vi "מסך ייצור 2 8.11.vi"(1 "Order":string[](array[string])) -> ()   [LabVIEW 2013]
uses:
  <vilib>/Utility/file.llb/Read From Spreadsheet File (string).vi
  Global 3.vi
  <vilib>/Utility/file.llb/Write To Spreadsheet File (string).vi
panel:
  out "element 2":string
  out "element":string
  out "row":i32
  out "output string":string
  out "decimal integer string":string[](array[string])
  out "size(s)":i32[](array[numeric])
  in  "v ok":bool
  out "Boolean 7":bool
  out "Boolean 6":bool
  out "Boolean 8":bool
  out "orders":string[][](array[string])
  out "int 9":dbl
  out "N itertion 9":dbl
  out "x/y 9":dbl
  out "int 8":dbl
  out "N itertion 8":dbl
  out "x/y 8":dbl
  out "x/y 7":dbl
  out "N itertion 7":dbl
  out "int 7":dbl
  out "int 6":dbl
  out "N itertion 6":dbl
  out "x/y 6":dbl
  out "int 5":dbl
  out "N itertion 5":dbl
  out "x/y 5":dbl
  out "x/y 4":dbl
  out "N itertion 4":dbl
  out "int 4":dbl
  out "Boolean 5":bool
  out "Boolean 4":bool
  out "Boolean 3":bool
  out "Boolean 2":bool
  out "Boolean":bool
  out "ML INT":dbl
  out "x/y 3":dbl
  out "N itertion 3":dbl
  out "int 3":dbl
  out "x/y 2":dbl
  out "N itertion 2":dbl
  out "int 2":dbl
  out "int":dbl
  out "N itertion":dbl
  out "x/y":dbl
  out "camot":dbl
  out "CAMOT":string
  out "ML":string
  out "Virus C":dbl(slide) scale=0.0..80.0
  out "Virus B":dbl(slide) scale=0.0..80.0
  out "Virus A":dbl(slide) scale=0.0..80.0
  out "HISON":string
  in  "EXIT":bool
  out "bottels ready":dbl(slide)
  out "Production Tank":dbl(slide) scale=0.0..100.0
  in  "start":bool
  out "Water":dbl(slide) scale=0.0..50.0
  out "Classifier material":dbl(slide) scale=0.0..25.0
  out "status":string
  # "Fider"
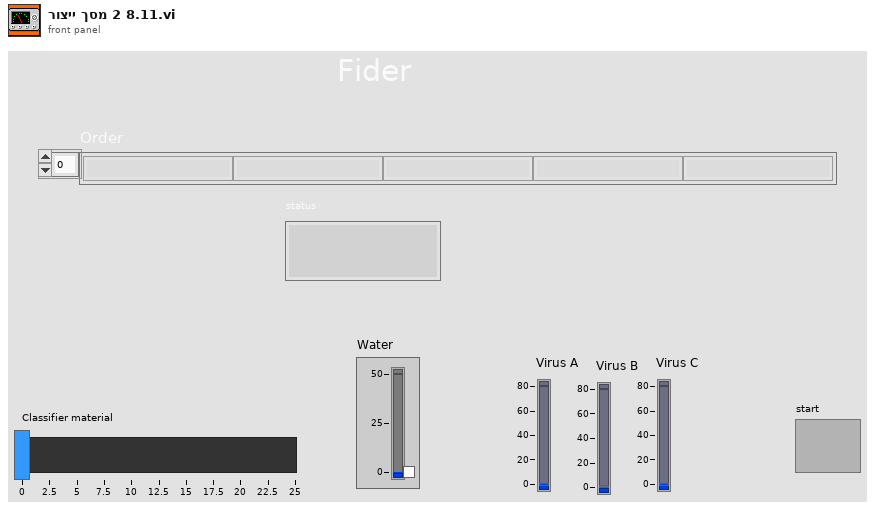
[diagram p1: front panel]
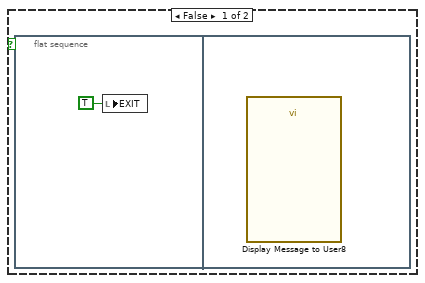
[diagram p3: hidden frame]
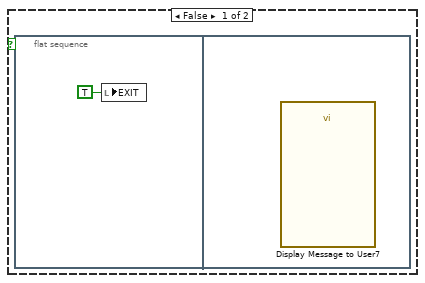
[diagram p5: hidden frame]
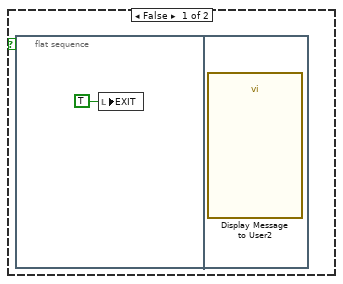
[diagram p7: hidden frame]
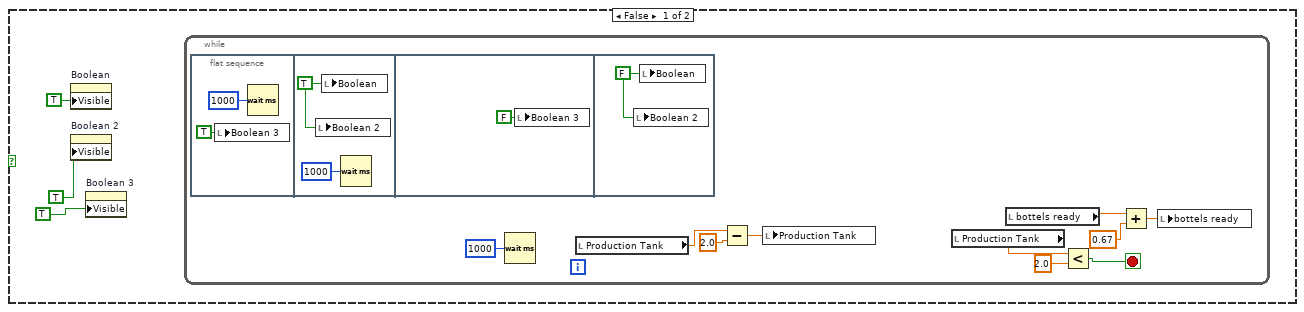
[diagram p10: hidden frame]
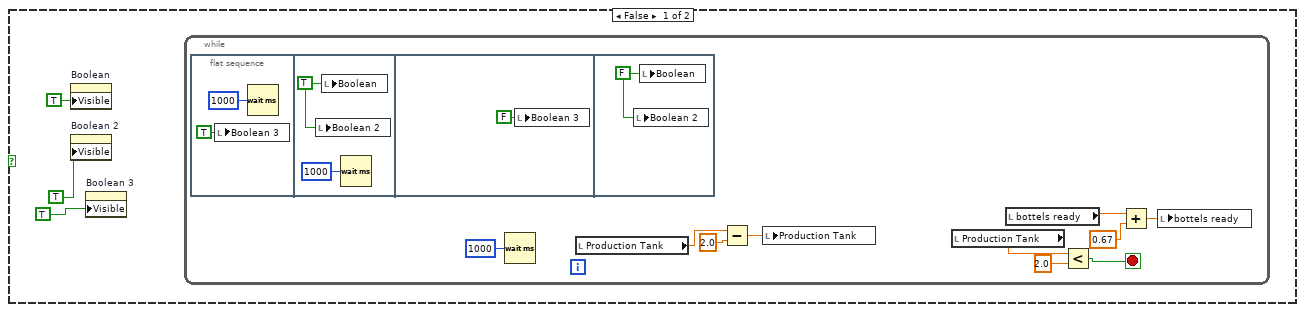
[diagram p12: hidden frame]
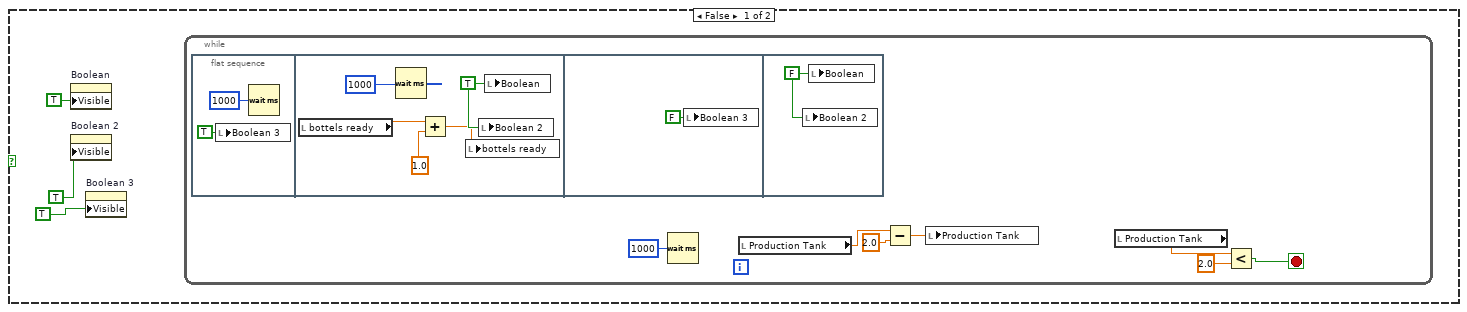
[diagram p14: hidden frame]
diagram:
  n1 = flat-sequence {
    frame #0 {
      n2 = local write "v ok"(FALSE ("v ok")) -> ()
      n3 = local write "EXIT"(FALSE ("EXIT")) -> ()
      n4 = local write "start"(FALSE ("start")) -> ()
    }
    frame #1 {
      n5 = while {
        stop <- "EXIT" stop-if-true
        n6 = local read "Order"() -> (w42:string[])
        n7 = property on="Classifier material" class="Slide (strict)"("Visible"=TRUE) -> ()  [unwired: 2 in, 2 out]
        n8 = global read "Global 3.vi" "Virus C"() -> (→"Virus C":dbl)
        n9 = property on="Boolean 4" class="Bool (strict)"("Visible"=FALSE) -> ()  [unwired: 2 in, 2 out]
        n10 = property on="Boolean" class="Bool (strict)"("Visible"=FALSE) -> ()  [unwired: 2 in, 2 out]
        n11 = property on="Boolean 2" class="Bool (strict)"("Visible"=FALSE) -> ()  [unwired: 2 in, 2 out]
        n12 = property on="Boolean 5" class="Bool (strict)"("Visible"=FALSE) -> ()  [unwired: 2 in, 2 out]
        n13 = property on="Boolean 3" class="Bool (strict)"("Visible"=FALSE) -> ()  [unwired: 2 in, 2 out]
        n14 = local read "Order"() -> (w41:string[])
        n15 = property on="Production Tank" class="Slide (strict)"("Blinking"=FALSE) -> ()  [unwired: 2 in, 2 out]
        n16 = property on="Production Tank" class="Slide (strict)"("Visible"=FALSE) -> ()  [unwired: 2 in, 2 out]
        n17 = Index Array(array=w42, index=2) -> (element=→"HISON":string)
        n18 = property on="bottels ready" class="Slide (strict)"("Visible"=FALSE) -> ()  [unwired: 2 in, 2 out]
        n19 = property on="Water" class="Slide (strict)"("Visible"=TRUE) -> ()  [unwired: 2 in, 2 out]
        n20 = global read "Global 3.vi" "Virus B"() -> (→"Virus B":dbl)
        n21 = local read "decimal integer string"() -> (w7:string[])
        n22 = Index Array(array=w41, index=4) -> (element=→"CAMOT":string)
        n23 = property on="Virus A" class="Slide (strict)"("Visible"=TRUE) -> ()  [unwired: 2 in, 2 out]
        n24 = property on="Virus B" class="Slide (strict)"("Visible"=TRUE) -> ()  [unwired: 2 in, 2 out]
        n25 = local read "Order"() -> (w40:string[])
        n26 = Current VI's Path() -> (path=w18:path)
        n27 = local read "orders"() -> (w10:string[][])
        n28 = property on="Virus C" class="Slide (strict)"("Visible"=TRUE) -> ()  [unwired: 2 in, 2 out]
        n29 = Strip Path(path=w18) -> (stripped path=w17:path)  [unwired: 1 out]
        n30 = local read "CAMOT"() -> (w22:string)
        n31 = global read "Global 3.vi" "Virus A"() -> (→"Virus A":dbl)
        n32 = global read "Global 3.vi" "Classifier material"() -> (→"Classifier material":dbl)
        n33 = Index String Array(1:0 ("index"), 2:w7) -> (0:w5:string)  [unwired: 1 in]
        "output string" <- w5
        n34 = local read "camot"() -> (w21:dbl)
        n35 = Index Array(array=w40, index=3) -> (element=→"ML":string)
        n36 = Build Path(base path=w17, name or relative path="order list.xls") -> (appended path=w16:path)
        n37 = Array Size(array=w10) -> (size(s)=w9:i32[])
        "size(s)" <- w9
        n38 = Fract/Exp String To Number(string=w22) -> (number=→"camot":dbl)  [unwired: 3 in, 1 out]
        n39 = global read "Global 3.vi" "Water"() -> (→"Water":dbl)
        n40 = Decimal String To Number(string=w5) -> (number=→"row":i32)  [unwired: 2 in, 1 out]
        n41 = property on="bottels ready" class="Slide (strict)"("Scale.Maximum"=w21) -> ()  [unwired: 2 in, 2 out]
        n42 = call-poly <vilib>:"Read From Spreadsheet File.vi"("file path (dialog if empty)"=w16) -> ("all rows"=→"orders":string[][])  [unwired: 6 in, 4 out]
        n43 = local read "ML"() -> (w39:string)
        n44 = Number To Decimal String(number=w9) -> (decimal integer string=→"decimal integer string":string[])  [unwired: 1 in]
        n45 = Fract/Exp String To Number(string=w39) -> (number=→"ML INT":dbl)  [unwired: 3 in, 1 out]
        n46 = flat-sequence {
          frame #0 {
            n47 = local read "HISON"() -> (w59:string)
            n48 = local read "HISON"() -> (w57:string)
            n49 = Equal?(x=w59, y="Jaundice") -> (x = y?=w60:bool)
            n50 = local read "HISON"() -> (w54:string)
            n51 = case shown="True" w60 {
              frame False {
              }
              frame True {
                n52 = local read "ML INT"() -> (w76:dbl)
                n53 = local read "ML INT"() -> (w71:dbl)
                n54 = local read "ML INT"() -> (w68:dbl)
                n55 = local read "Classifier material"() -> (w81:dbl)
                n56 = local read "Virus C"() -> (w83:dbl)
                n57 = local read "Water"() -> (w82:dbl)
                n58 = Multiply(x=w76, y=0.08) -> (x*y=w77:dbl)
                n59 = Multiply(x=w71, y=0.9) -> (x*y=w70:dbl)
                n60 = Multiply(x=w68, y=0.02) -> (x*y=w69:dbl)
                n61 = local read "camot"() -> (w74:dbl)
                n62 = local read "camot"() -> (w73:dbl)
                n63 = local read "camot"() -> (w66:dbl)
                n64 = Multiply(x=w74, y=w77) -> (x*y=w78:dbl)
                n65 = Greater Or Equal?(x=w81, y=w78) -> (x >= y?=w62:bool)
                n66 = Multiply(x=w73, y=w70) -> (x*y=w79:dbl)
                n67 = Greater Or Equal?(x=w82, y=w79) -> (x >= y?=w63:bool)
                n68 = Multiply(x=w66, y=w69) -> (x*y=w80:dbl)
                n69 = And(x=w62, y=w63) -> (x .and. y?=w64:bool)
                n70 = Greater Or Equal?(x=w83, y=w80) -> (x >= y?=w65:bool)
                n71 = And(x=w64, y=w65) -> (x .and. y?=w61:bool)
                n72 = case shown="True" w61 {
                  frame False {
                    n73 = flat-sequence {
                      frame #0 {
                        n74 = local write "EXIT"(TRUE ("EXIT")) -> ()
                      }
                      frame #1 {
                        n75 = call "Display Message to User8"() -> ()  [unwired: 10 in, 2 out]
                      }
                    }
                  }
                  frame True {
                    n76 = property on="start" class="Bool (strict)"("Visible"=TRUE) -> ()  [unwired: 2 in, 2 out]
                    "Boolean 8" <- TRUE ("Boolean 6")
                  }
                }
              }
            }
            n77 = Equal?(x=w57, y="Influenza") -> (x = y?=w58:bool)
            n78 = case shown="True" w58 {
              frame False {
              }
              frame True {
                n79 = local read "ML INT"() -> (w104:dbl)
                n80 = local read "ML INT"() -> (w99:dbl)
                n81 = local read "Classifier material"() -> (w107:dbl)
                n82 = local read "ML INT"() -> (w93:dbl)
                n83 = Multiply(x=w104, y=0.81) -> (x*y=w105:dbl)
                n84 = Multiply(x=w99, y=0.15) -> (x*y=w100:dbl)
                n85 = local read "camot"() -> (w102:dbl)
                n86 = local read "camot"() -> (w97:dbl)
                n87 = local read "Virus B"() -> (w109:dbl)
                n88 = local read "camot"() -> (w95:dbl)
                n89 = Multiply(x=w102, y=w105) -> (x*y=w106:dbl)
                n90 = Multiply(x=w97, y=w100) -> (x*y=w101:dbl)
                n91 = Multiply(x=0.04 ("y"), y=w93) -> (x*y=w92:dbl)
                n92 = local read "Water"() -> (w108:dbl)
                n93 = Greater Or Equal?(x=w108, y=w101) -> (x >= y?=w89:bool)
                n94 = Multiply(x=w95, y=w92) -> (x*y=w96:dbl)
                n95 = Greater Or Equal?(x=w109, y=w106) -> (x >= y?=w91:bool)
                n96 = And(x=w89, y=w91) -> (x .and. y?=w90:bool)
                n97 = Greater Or Equal?(x=w107, y=w96) -> (x >= y?=w88:bool)
                n98 = And(x=w88, y=w90) -> (x .and. y?=w87:bool)
                n99 = case shown="True" w87 {
                  frame False {
                    n100 = flat-sequence {
                      frame #0 {
                        n101 = local write "EXIT"(TRUE ("EXIT")) -> ()
                      }
                      frame #1 {
                        n102 = call "Display Message to User7"() -> ()  [unwired: 10 in, 2 out]
                      }
                    }
                  }
                  frame True {
                    n103 = property on="start" class="Bool (strict)"("Visible"=TRUE) -> ()  [unwired: 2 in, 2 out]
                    "Boolean 7" <- TRUE ("Boolean 6")
                  }
                }
              }
            }
            n104 = Equal?(x=w54, y="COVID-19") -> (x = y?=w55:bool)
            n105 = case shown="True" w55 {
              frame False {
              }
              frame True {
                n106 = local read "ML INT"() -> (w129:dbl)
                n107 = local read "ML INT"() -> (w119:dbl)
                n108 = local read "ML INT"() -> (w125:dbl)
                n109 = local read "Classifier material"() -> (w133:dbl)
                n110 = local read "camot"() -> (w131:dbl)
                n111 = Multiply(x=0.05 ("y"), y=w129) -> (x*y=w128:dbl)
                n112 = local read "Water"() -> (w134:dbl)
                n113 = local read "camot"() -> (w121:dbl)
                n114 = local read "camot"() -> (w123:dbl)
                n115 = Multiply(x=0.22 ("y"), y=w119) -> (x*y=w118:dbl)
                n116 = Multiply(x=0.73 ("y"), y=w125) -> (x*y=w126:dbl)
                n117 = Multiply(x=w131, y=w128) -> (x*y=w132:dbl)
                n118 = Greater Or Equal?(x=w133, y=w132) -> (x >= y?=w114:bool)
                n119 = Multiply(x=w121, y=w118) -> (x*y=w122:dbl)
                n120 = Multiply(x=w123, y=w126) -> (x*y=w127:dbl)
                n121 = Greater Or Equal?(x=w134, y=w127) -> (x >= y?=w115:bool)
                n122 = And(x=w114, y=w115) -> (x .and. y?=w117:bool)
                n123 = local read "Virus A"() -> (w135:dbl)
                n124 = Greater Or Equal?(x=w135, y=w122) -> (x >= y?=w116:bool)
                n125 = And(x=w117, y=w116) -> (x .and. y?=w113:bool)
                n126 = case shown="True" w113 {
                  frame False {
                    n127 = flat-sequence {
                      frame #0 {
                        n128 = local write "EXIT"(TRUE ("EXIT")) -> ()
                      }
                      frame #1 {
                        n129 = call "Display Message to User2"() -> ()  [unwired: 10 in, 2 out]
                      }
                    }
                  }
                  frame True {
                    n130 = property on="start" class="Bool (strict)"("Visible"=TRUE) -> ()  [unwired: 2 in, 2 out]
                    "Boolean 6" <- TRUE ("Boolean 6")
                  }
                }
              }
            }
          }
          frame #1 {
            n131 = case shown="True" "start" {
              frame False {
              }
              frame True {
                n132 = local read "Boolean 7"() -> (w141:bool)
                n133 = local read "Boolean 8"() -> (w140:bool)
                n134 = case shown="True" w141 {
                  frame False {
                  }
                  frame True {
                    n135 = flat-sequence {
                      frame #0 {
                        n136 = property on="Production Tank" class="Slide (strict)"("Visible"=TRUE) -> ()  [unwired: 2 in, 2 out]
                        n137 = property on="start" class="Bool (strict)"("Visible"=FALSE) -> ()  [unwired: 2 in, 2 out]
                        n138 = local write "start"(FALSE ("start")) -> ()
                      }
                      frame #1 {
                        n139 = local read "ML INT"() -> (w335:dbl)
                        n140 = local read "N itertion 4"() -> (w337:dbl)
                        n141 = Multiply(x=0.04 ("y"), y=w335) -> (x*y=w334:dbl)
                        n142 = local read "x/y 4"() -> (w340:dbl)
                        n143 = local read "camot"() -> (w342:dbl)
                        n144 = Round Toward -Infinity(1:w340) -> (0:→"N itertion 4":dbl)
                        n145 = Multiply(x=w342, y=w334) -> (x*y=w343:dbl)
                        n146 = Multiply(x=w337, y=2.0) -> (x*y=→"int 4":dbl)
                        n147 = Divide(x=w343, y=2.0) -> (x/y=→"x/y 4":dbl)
                      }
                      frame #2 {
                        n148 = local read "N itertion 4"() -> (w346:dbl)
                        n149 = for {
                          N: w346 -> [_]
                          n150 = local read "Classifier material"() -> (w354:dbl)
                          n151 = local read "Production Tank"() -> (w352:dbl)
                          n152 = Wait (ms)(milliseconds to wait=u32 1000) -> ()  [unwired: 1 out]
                          n153 = Add(x=w352, y=2.0) -> (x+y=w351:dbl)
                          n154 = Subtract(x=w354, y=2.0) -> (x-y=w353:dbl)
                          n155 = local write "Production Tank"(w351) -> ()
                          n156 = local write "Classifier material"(w353) -> ()
                          n157 = local write "status"("Addind Classified material" ("status")) -> ()
                        }
                      }
                      frame #3 {
                        n158 = local read "ML INT"() -> (w358:dbl)
                        n159 = local read "ML INT"() -> (w359:dbl)
                        n160 = local write "status"("Addind Classified material" ("status")) -> ()
                        n161 = Multiply(x=0.04 ("y"), y=w358) -> (x*y=w356:dbl)
                        n162 = Multiply(x=0.04 ("y"), y=w359) -> (x*y=w355:dbl)
                        n163 = local read "camot"() -> (w372:dbl)
                        n164 = local read "camot"() -> (w365:dbl)
                        n165 = Multiply(x=w372, y=w356) -> (x*y=w371:dbl)
                        n166 = Multiply(x=w365, y=w355) -> (x*y=w364:dbl)
                        n167 = local read "int 4"() -> (w370:dbl)
                        n168 = local read "int 4"() -> (w363:dbl)
                        n169 = Subtract(x=w371, y=w370) -> (x-y=w369:dbl)
                        n170 = Subtract(x=w364, y=w363) -> (x-y=w366:dbl)
                        n171 = local read "Classifier material"() -> (w373:dbl)
                        n172 = local read "Production Tank"() -> (w367:dbl)
                        n173 = Subtract(x=w373, y=w369) -> (x-y=w374:dbl)
                        n174 = Add(x=w367, y=w366) -> (x+y=w368:dbl)
                        n175 = local write "Classifier material"(w374) -> ()
                        n176 = local write "Production Tank"(w368) -> ()
                        n177 = Wait (ms)(milliseconds to wait=u32 1000) -> ()  [unwired: 1 out]
                      }
                      frame #4 {
                        n178 = local read "ML INT"() -> (w376:dbl)
                        n179 = Multiply(x=w376, y=0.15) -> (x*y=w375:dbl)
                        n180 = local read "camot"() -> (w381:dbl)
                        n181 = Multiply(x=w381, y=w375) -> (x*y=w380:dbl)
                        n182 = Divide(x=w380, y=2.0) -> (x/y=→"x/y 5":dbl)
                      }
                      frame #5 {
                        n183 = local read "x/y 5"() -> (w383:dbl)
                        n184 = Round Toward -Infinity(1:w383) -> (0:→"N itertion 5":dbl)
                      }
                      frame #6 {
                        n185 = local read "N itertion 5"() -> (w384:dbl)
                        n186 = Multiply(x=w384, y=2.0) -> (x*y=→"int 5":dbl)
                      }
                      frame #7 {
                        n187 = local read "N itertion 5"() -> (w387:dbl)
                        n188 = for {
                          N: w387 -> [_]
                          n189 = local read "Water"() -> (w394:dbl)
                          n190 = Wait (ms)(milliseconds to wait=u32 1000) -> ()  [unwired: 1 out]
                          n191 = local read "Production Tank"() -> (w388:dbl)
                          n192 = Subtract(x=w394, y=2.0) -> (x-y=w395:dbl)
                          n193 = local write "Water"(w395) -> ()
                          n194 = local write "status"("Addind Water" ("status")) -> ()
                          n195 = Add(x=w388, y=2.0) -> (x+y=w389:dbl)
                          n196 = local write "Production Tank"(w389) -> ()
                        }
                      }
                      frame #8 {
                        n197 = local read "ML INT"() -> (w399:dbl)
                        n198 = local read "ML INT"() -> (w401:dbl)
                        n199 = Multiply(x=w399, y=0.15) -> (x*y=w396:dbl)
                        n200 = Multiply(x=w401, y=0.15) -> (x*y=w397:dbl)
                        n201 = local read "camot"() -> (w411:dbl)
                        n202 = local read "camot"() -> (w406:dbl)
                        n203 = Multiply(x=w411, y=w396) -> (x*y=w412:dbl)
                        n204 = Multiply(x=w406, y=w397) -> (x*y=w407:dbl)
                        n205 = local read "int 5"() -> (w410:dbl)
                        n206 = local read "int 5"() -> (w402:dbl)
                        n207 = Subtract(x=w412, y=w410) -> (x-y=w413:dbl)
                        n208 = Subtract(x=w407, y=w402) -> (x-y=w405:dbl)
                        n209 = local read "Production Tank"() -> (w404:dbl)
                        n210 = local read "Water"() -> (w408:dbl)
                        n211 = Subtract(x=w408, y=w413) -> (x-y=w409:dbl)
                        n212 = Add(x=w404, y=w405) -> (x+y=w403:dbl)
                        n213 = local write "Production Tank"(w403) -> ()
                        n214 = local write "Water"(w409) -> ()
                        n215 = Wait (ms)(milliseconds to wait=u32 1000) -> ()  [unwired: 1 out]
                      }
                      frame #9 {
                        n216 = local read "ML INT"() -> (w416:dbl)
                        n217 = Multiply(x=w416, y=0.81) -> (x*y=w415:dbl)
                        n218 = local read "camot"() -> (w421:dbl)
                        n219 = Multiply(x=w421, y=w415) -> (x*y=w420:dbl)
                        n220 = Divide(x=w420, y=2.0) -> (x/y=→"x/y 6":dbl)
                      }
                      frame #10 {
                        n221 = local read "x/y 6"() -> (w423:dbl)
                        n222 = Round Toward -Infinity(1:w423) -> (0:→"N itertion 6":dbl)
                      }
                      frame #11 {
                        n223 = local read "N itertion 6"() -> (w424:dbl)
                        n224 = Multiply(x=w424, y=2.0) -> (x*y=→"int 6":dbl)
                      }
                      frame #12 {
                        n225 = local read "N itertion 6"() -> (w427:dbl)
                        n226 = for {
                          N: w427 -> [_]
                          n227 = local read "Virus B"() -> (w428:dbl)
                          n228 = local read "Production Tank"() -> (w431:dbl)
                          n229 = Wait (ms)(milliseconds to wait=u32 1000) -> ()  [unwired: 1 out]
                          n230 = Subtract(x=w428, y=2.0) -> (x-y=w429:dbl)
                          n231 = local write "status"("Addind Virus B" ("status")) -> ()
                          n232 = local write "Virus B"(w429) -> ()
                          n233 = Add(x=w431, y=2.0) -> (x+y=w432:dbl)
                          n234 = local write "Production Tank"(w432) -> ()
                        }
                      }
                      frame #13 {
                        n235 = local read "ML INT"() -> (w440:dbl)
                        n236 = local read "ML INT"() -> (w443:dbl)
                        n237 = Multiply(x=w440, y=0.81) -> (x*y=w438:dbl)
                        n238 = Multiply(x=w443, y=0.81) -> (x*y=w441:dbl)
                        n239 = local read "camot"() -> (w451:dbl)
                        n240 = local read "camot"() -> (w449:dbl)
                        n241 = Multiply(x=w451, y=w438) -> (x*y=w450:dbl)
                        n242 = Multiply(x=w449, y=w441) -> (x*y=w448:dbl)
                        n243 = local read "int 6"() -> (w444:dbl)
                        n244 = local read "int 6"() -> (w445:dbl)
                        n245 = Subtract(x=w450, y=w444) -> (x-y=w452:dbl)
                        n246 = Subtract(x=w448, y=w445) -> (x-y=w447:dbl)
                        n247 = local read "Production Tank"() -> (w453:dbl)
                        n248 = local read "Virus B"() -> (w437:dbl)
                        n249 = Add(x=w453, y=w452) -> (x+y=w454:dbl)
                        n250 = Subtract(x=w437, y=w447) -> (x-y=w436:dbl)
                        n251 = local write "Production Tank"(w454) -> ()
                        n252 = local write "Virus B"(w436) -> ()
                        n253 = Wait (ms)(milliseconds to wait=u32 1000) -> ()  [unwired: 1 out]
                      }
                      frame #14 {
                        n254 = Wait (ms)(milliseconds to wait=u32 17000) -> ()  [unwired: 1 out]
                        n255 = property on="Production Tank" class="Slide (strict)"("Blinking"=TRUE) -> ()  [unwired: 2 in, 2 out]
                        n256 = local write "status"("Quality Control" ("status")) -> ()
                      }
                      frame #15 {
                        n257 = local read "ML INT"() -> (w460:dbl)
                        n258 = property on="Production Tank" class="Slide (strict)"("Blinking"=FALSE) -> ()  [unwired: 2 in, 2 out]
                        n259 = Equal?(x=w460, y=5.0) -> (x = y?=w458:bool)
                        n260 = property on="bottels ready" class="Slide (strict)"("Visible"=TRUE) -> ()  [unwired: 2 in, 2 out]
                        n261 = case shown="True" w458 {
                          frame False {
                            n262 = property on="Boolean" class="Bool (strict)"("Visible"=TRUE) -> ()  [unwired: 2 in, 2 out]
                            n263 = property on="Boolean 2" class="Bool (strict)"("Visible"=TRUE) -> ()  [unwired: 2 in, 2 out]
                            n264 = property on="Boolean 3" class="Bool (strict)"("Visible"=TRUE) -> ()  [unwired: 2 in, 2 out]
                            n265 = while {
                              stop <- w475 stop-if-true
                              n266 = flat-sequence {
                                frame #0 {
                                n267 = local write "Boolean 3"(TRUE ("Boolean 3")) -> ()
                                n268 = Wait (ms)(milliseconds to wait=u32 1000) -> ()  [unwired: 1 out]
                                }
                                frame #1 {
                                w485 = TRUE ("Boolean")
                                n269 = local write "Boolean 2"(w485) -> ()
                                n270 = local write "Boolean"(w485) -> ()
                                n271 = Wait (ms)(milliseconds to wait=u32 1000) -> ()  [unwired: 1 out]
                                }
                                frame #2 {
                                n272 = local write "Boolean 3"(FALSE ("Boolean 3")) -> ()
                                }
                                frame #3 {
                                w487 = FALSE ("Boolean")
                                n273 = local write "Boolean 2"(w487) -> ()
                                n274 = local write "Boolean"(w487) -> ()
                                }
                              }
                              n275 = Wait (ms)(milliseconds to wait=u32 1000) -> ()  [unwired: 1 out]
                              n276 = local read "Production Tank"() -> (w481:dbl)
                              n277 = Subtract(x=w481, y=2.0) -> (x-y=w480:dbl)
                              n278 = local write "Production Tank"(w480) -> ()
                              n279 = local read "Production Tank"() -> (w476:dbl)
                              n280 = local read "bottels ready"() -> (w472:dbl)
                              n281 = Less?(x=w476, y=2.0) -> (x < y?=w475:bool)
                              n282 = Add(x=w472, y=0.67) -> (x+y=w473:dbl)
                              n283 = local write "bottels ready"(w473) -> ()
                            }
                          }
                          frame True {
                            n284 = property on="Boolean 5" class="Bool (strict)"("Visible"=TRUE) -> ()  [unwired: 2 in, 2 out]
                            n285 = property on="Boolean" class="Bool (strict)"("Visible"=TRUE) -> ()  [unwired: 2 in, 2 out]
                            n286 = property on="Boolean 2" class="Bool (strict)"("Visible"=TRUE) -> ()  [unwired: 2 in, 2 out]
                            n287 = property on="Boolean 4" class="Bool (strict)"("Visible"=TRUE) -> ()  [unwired: 2 in, 2 out]
                            n288 = property on="Boolean 3" class="Bool (strict)"("Visible"=TRUE) -> ()  [unwired: 2 in, 2 out]
                            n289 = while {
                              stop <- w494 stop-if-true
                              n290 = flat-sequence {
                                frame #0 {
                                n291 = local write "Boolean 5"(TRUE ("Boolean 5")) -> ()
                                n292 = Wait (ms)(milliseconds to wait=u32 500) -> ()  [unwired: 1 out]
                                }
                                frame #1 {
                                w506 = TRUE ("Boolean 3")
                                n293 = local write "Boolean 4"(w506) -> ()
                                n294 = local write "Boolean 3"(w506) -> ()
                                n295 = Wait (ms)(milliseconds to wait=u32 500) -> ()  [unwired: 1 out]
                                }
                                frame #2 {
                                w508 = TRUE ("Boolean")
                                n296 = local write "Boolean 2"(w508) -> ()
                                n297 = local write "Boolean"(w508) -> ()
                                n298 = Wait (ms)(milliseconds to wait=u32 500) -> ()  [unwired: 1 out]
                                }
                                frame #3 {
                                n299 = local write "Boolean 5"(FALSE ("Boolean 5")) -> ()
                                }
                                frame #4 {
                                w510 = FALSE ("Boolean 3")
                                n300 = local write "Boolean 4"(w510) -> ()
                                n301 = local write "Boolean 3"(w510) -> ()
                                }
                                frame #5 {
                                w511 = FALSE ("Boolean")
                                n302 = local write "Boolean 2"(w511) -> ()
                                n303 = local write "Boolean"(w511) -> ()
                                }
                              }
                              n304 = Wait (ms)(milliseconds to wait=u32 1000) -> ()  [unwired: 1 out]
                              n305 = local read "Production Tank"() -> (w502:dbl)
                              n306 = Subtract(x=w502, y=2.0) -> (x-y=w501:dbl)
                              n307 = local write "Production Tank"(w501) -> ()
                              n308 = local read "bottels ready"() -> (w498:dbl)
                              n309 = local read "Production Tank"() -> (w493:dbl)
                              n310 = Add(x=w498, y=0.4) -> (x+y=w497:dbl)
                              n311 = Less?(x=w493, y=2.0) -> (x < y?=w494:bool)
                              n312 = local write "bottels ready"(w497) -> ()
                            }
                          }
                        }
                        n313 = local write "status"("Filling Bottels" ("status")) -> ()
                        n314 = property on="Classifier material" class="Slide (strict)"("Visible"=FALSE) -> ()  [unwired: 2 in, 2 out]
                        n315 = property on="Water" class="Slide (strict)"("Visible"=FALSE) -> ()  [unwired: 2 in, 2 out]
                        n316 = property on="Virus A" class="Slide (strict)"("Visible"=FALSE) -> ()  [unwired: 2 in, 2 out]
                        n317 = property on="Virus B" class="Slide (strict)"("Visible"=FALSE) -> ()  [unwired: 2 in, 2 out]
                        n318 = property on="Virus C" class="Slide (strict)"("Visible"=FALSE) -> ()  [unwired: 2 in, 2 out]
                      }
                      frame #16 {
                        n319 = local read "Classifier material"() -> (w513:dbl)
                        n320 = local write "v ok"(TRUE ("v ok")) -> ()
                        n321 = local write "EXIT"(TRUE ("EXIT")) -> ()
                        n322 = local read "Virus B"() -> (w516:dbl)
                        n323 = local read "Virus C"() -> (w517:dbl)
                        n324 = local read "Virus A"() -> (w515:dbl)
                        n325 = local read "Water"() -> (w514:dbl)
                        n326 = global write "Global 3.vi" "Classifier material"(w513) -> ()
                        n327 = global write "Global 3.vi" "Virus C"(w517) -> ()
                        n328 = global write "Global 3.vi" "Virus B"(w516) -> ()
                        n329 = global write "Global 3.vi" "Virus A"(w515) -> ()
                        n330 = global write "Global 3.vi" "Water"(w514) -> ()
                      }
                    }
                  }
                }
                n331 = local read "Boolean 6"() -> (w142:bool)
                n332 = case shown="True" w140 {
                  frame False {
                  }
                  frame True {
                    n333 = flat-sequence {
                      frame #0 {
                        n334 = local write "start"(FALSE ("start")) -> ()
                        n335 = property on="start" class="Bool (strict)"("Visible"=FALSE) -> ()  [unwired: 2 in, 2 out]
                        n336 = property on="Production Tank" class="Slide (strict)"("Visible"=TRUE) -> ()  [unwired: 2 in, 2 out]
                      }
                      frame #1 {
                        n337 = local read "ML INT"() -> (w147:dbl)
                        n338 = local read "N itertion 7"() -> (w149:dbl)
                        n339 = Multiply(x=0.08 ("y"), y=w147) -> (x*y=w146:dbl)
                        n340 = local read "x/y 7"() -> (w152:dbl)
                        n341 = local read "camot"() -> (w154:dbl)
                        n342 = Round Toward -Infinity(1:w152) -> (0:→"N itertion 7":dbl)
                        n343 = Multiply(x=w154, y=w146) -> (x*y=w155:dbl)
                        n344 = Multiply(x=w149, y=2.0) -> (x*y=→"int 7":dbl)
                        n345 = Divide(x=w155, y=2.0) -> (x/y=→"x/y 7":dbl)
                      }
                      frame #2 {
                        n346 = local read "N itertion 7"() -> (w158:dbl)
                        n347 = for {
                          N: w158 -> [_]
                          n348 = local read "Classifier material"() -> (w166:dbl)
                          n349 = local read "Production Tank"() -> (w164:dbl)
                          n350 = Wait (ms)(milliseconds to wait=u32 1000) -> ()  [unwired: 1 out]
                          n351 = Add(x=w164, y=2.0) -> (x+y=w163:dbl)
                          n352 = Subtract(x=w166, y=2.0) -> (x-y=w165:dbl)
                          n353 = local write "Production Tank"(w163) -> ()
                          n354 = local write "Classifier material"(w165) -> ()
                          n355 = local write "status"("Addind Classified material" ("status")) -> ()
                        }
                      }
                      frame #3 {
                        n356 = local read "ML INT"() -> (w170:dbl)
                        n357 = local read "ML INT"() -> (w171:dbl)
                        n358 = local write "status"("Addind Classified material" ("status")) -> ()
                        n359 = Multiply(x=0.08 ("y"), y=w170) -> (x*y=w168:dbl)
                        n360 = Multiply(x=0.08 ("y"), y=w171) -> (x*y=w167:dbl)
                        n361 = local read "camot"() -> (w184:dbl)
                        n362 = local read "camot"() -> (w177:dbl)
                        n363 = Multiply(x=w184, y=w168) -> (x*y=w183:dbl)
                        n364 = Multiply(x=w177, y=w167) -> (x*y=w176:dbl)
                        n365 = local read "int 7"() -> (w182:dbl)
                        n366 = local read "int 7"() -> (w175:dbl)
                        n367 = Subtract(x=w183, y=w182) -> (x-y=w181:dbl)
                        n368 = Subtract(x=w176, y=w175) -> (x-y=w178:dbl)
                        n369 = local read "Classifier material"() -> (w185:dbl)
                        n370 = local read "Production Tank"() -> (w179:dbl)
                        n371 = Subtract(x=w185, y=w181) -> (x-y=w186:dbl)
                        n372 = Add(x=w179, y=w178) -> (x+y=w180:dbl)
                        n373 = local write "Classifier material"(w186) -> ()
                        n374 = local write "Production Tank"(w180) -> ()
                        n375 = Wait (ms)(milliseconds to wait=u32 1000) -> ()  [unwired: 1 out]
                      }
                      frame #4 {
                        n376 = local read "ML INT"() -> (w188:dbl)
                        n377 = Multiply(x=w188, y=0.02) -> (x*y=w187:dbl)
                        n378 = local read "camot"() -> (w193:dbl)
                        n379 = Multiply(x=w193, y=w187) -> (x*y=w192:dbl)
                        n380 = Divide(x=w192, y=2.0) -> (x/y=→"x/y 8":dbl)
                      }
                      frame #5 {
                        n381 = local read "x/y 8"() -> (w195:dbl)
                        n382 = Round Toward -Infinity(1:w195) -> (0:→"N itertion 8":dbl)
                      }
                      frame #6 {
                        n383 = local read "N itertion 8"() -> (w196:dbl)
                        n384 = Multiply(x=w196, y=2.0) -> (x*y=→"int 8":dbl)
                      }
                      frame #7 {
                        n385 = local read "N itertion 8"() -> (w199:dbl)
                        n386 = for {
                          N: w199 -> [_]
                          n387 = local read "Water"() -> (w206:dbl)
                          n388 = Wait (ms)(milliseconds to wait=u32 1000) -> ()  [unwired: 1 out]
                          n389 = local read "Production Tank"() -> (w200:dbl)
                          n390 = Subtract(x=w206, y=2.0) -> (x-y=w207:dbl)
                          n391 = local write "Water"(w207) -> ()
                          n392 = local write "status"("Addind Water" ("status")) -> ()
                          n393 = Add(x=w200, y=2.0) -> (x+y=w201:dbl)
                          n394 = local write "Production Tank"(w201) -> ()
                        }
                      }
                      frame #8 {
                        n395 = local read "ML INT"() -> (w211:dbl)
                        n396 = local read "ML INT"() -> (w213:dbl)
                        n397 = Multiply(x=w211, y=0.02) -> (x*y=w208:dbl)
                        n398 = Multiply(x=w213, y=0.02) -> (x*y=w209:dbl)
                        n399 = local read "camot"() -> (w223:dbl)
                        n400 = local read "camot"() -> (w218:dbl)
                        n401 = Multiply(x=w223, y=w208) -> (x*y=w224:dbl)
                        n402 = Multiply(x=w218, y=w209) -> (x*y=w219:dbl)
                        n403 = local read "int 8"() -> (w222:dbl)
                        n404 = local read "int 8"() -> (w214:dbl)
                        n405 = Subtract(x=w224, y=w222) -> (x-y=w225:dbl)
                        n406 = Subtract(x=w219, y=w214) -> (x-y=w217:dbl)
                        n407 = local read "Production Tank"() -> (w216:dbl)
                        n408 = local read "Water"() -> (w220:dbl)
                        n409 = Subtract(x=w220, y=w225) -> (x-y=w221:dbl)
                        n410 = Add(x=w216, y=w217) -> (x+y=w215:dbl)
                        n411 = local write "Production Tank"(w215) -> ()
                        n412 = local write "Water"(w221) -> ()
                        n413 = Wait (ms)(milliseconds to wait=u32 1000) -> ()  [unwired: 1 out]
                      }
                      frame #9 {
                        n414 = local read "ML INT"() -> (w228:dbl)
                        n415 = Multiply(x=w228, y=0.9) -> (x*y=w227:dbl)
                        n416 = local read "camot"() -> (w233:dbl)
                        n417 = Multiply(x=w233, y=w227) -> (x*y=w232:dbl)
                        n418 = Divide(x=w232, y=2.0) -> (x/y=→"x/y 9":dbl)
                      }
                      frame #10 {
                        n419 = local read "x/y 9"() -> (w235:dbl)
                        n420 = Round Toward -Infinity(1:w235) -> (0:→"N itertion 9":dbl)
                      }
                      frame #11 {
                        n421 = local read "N itertion 9"() -> (w236:dbl)
                        n422 = Multiply(x=w236, y=2.0) -> (x*y=→"int 9":dbl)
                      }
                      frame #12 {
                        n423 = local read "N itertion 9"() -> (w239:dbl)
                        n424 = for {
                          N: w239 -> [_]
                          n425 = local read "Virus C"() -> (w240:dbl)
                          n426 = local read "Production Tank"() -> (w243:dbl)
                          n427 = Wait (ms)(milliseconds to wait=u32 1000) -> ()  [unwired: 1 out]
                          n428 = Subtract(x=w240, y=2.0) -> (x-y=w241:dbl)
                          n429 = local write "status"("Addind Virus B" ("status")) -> ()
                          n430 = local write "Virus C"(w241) -> ()
                          n431 = Add(x=w243, y=2.0) -> (x+y=w244:dbl)
                          n432 = local write "Production Tank"(w244) -> ()
                        }
                      }
                      frame #13 {
                        n433 = local read "ML INT"() -> (w252:dbl)
                        n434 = local read "ML INT"() -> (w255:dbl)
                        n435 = Multiply(x=w252, y=0.9) -> (x*y=w250:dbl)
                        n436 = Multiply(x=w255, y=0.9) -> (x*y=w253:dbl)
                        n437 = local read "camot"() -> (w263:dbl)
                        n438 = local read "camot"() -> (w261:dbl)
                        n439 = Multiply(x=w263, y=w250) -> (x*y=w262:dbl)
                        n440 = Multiply(x=w261, y=w253) -> (x*y=w260:dbl)
                        n441 = local read "int 9"() -> (w256:dbl)
                        n442 = local read "int 9"() -> (w257:dbl)
                        n443 = Subtract(x=w262, y=w256) -> (x-y=w264:dbl)
                        n444 = Subtract(x=w260, y=w257) -> (x-y=w259:dbl)
                        n445 = local read "Production Tank"() -> (w265:dbl)
                        n446 = local read "Virus C"() -> (w249:dbl)
                        n447 = Add(x=w265, y=w264) -> (x+y=w266:dbl)
                        n448 = Subtract(x=w249, y=w259) -> (x-y=w248:dbl)
                        n449 = local write "Production Tank"(w266) -> ()
                        n450 = local write "Virus C"(w248) -> ()
                        n451 = Wait (ms)(milliseconds to wait=u32 1000) -> ()  [unwired: 1 out]
                      }
                      frame #14 {
                        n452 = Wait (ms)(milliseconds to wait=u32 17000) -> ()  [unwired: 1 out]
                        n453 = property on="Production Tank" class="Slide (strict)"("Blinking"=TRUE) -> ()  [unwired: 2 in, 2 out]
                        n454 = local write "status"("Quality Control" ("status")) -> ()
                      }
                      frame #15 {
                        n455 = local read "ML INT"() -> (w274:dbl)
                        n456 = property on="Production Tank" class="Slide (strict)"("Blinking"=FALSE) -> ()  [unwired: 2 in, 2 out]
                        n457 = Equal?(x=w274, y=5.0) -> (x = y?=w272:bool)
                        n458 = case shown="True" w272 {
                          frame False {
                            n459 = property on="Boolean" class="Bool (strict)"("Visible"=TRUE) -> ()  [unwired: 2 in, 2 out]
                            n460 = property on="Boolean 2" class="Bool (strict)"("Visible"=TRUE) -> ()  [unwired: 2 in, 2 out]
                            n461 = property on="Boolean 3" class="Bool (strict)"("Visible"=TRUE) -> ()  [unwired: 2 in, 2 out]
                            n462 = while {
                              stop <- w287 stop-if-true
                              n463 = flat-sequence {
                                frame #0 {
                                n464 = local write "Boolean 3"(TRUE ("Boolean 3")) -> ()
                                n465 = Wait (ms)(milliseconds to wait=u32 1000) -> ()  [unwired: 1 out]
                                }
                                frame #1 {
                                w297 = TRUE ("Boolean")
                                n466 = local write "Boolean 2"(w297) -> ()
                                n467 = local write "Boolean"(w297) -> ()
                                n468 = Wait (ms)(milliseconds to wait=u32 1000) -> ()  [unwired: 1 out]
                                }
                                frame #2 {
                                n469 = local write "Boolean 3"(FALSE ("Boolean 3")) -> ()
                                }
                                frame #3 {
                                w299 = FALSE ("Boolean")
                                n470 = local write "Boolean 2"(w299) -> ()
                                n471 = local write "Boolean"(w299) -> ()
                                }
                              }
                              n472 = Wait (ms)(milliseconds to wait=u32 1000) -> ()  [unwired: 1 out]
                              n473 = local read "Production Tank"() -> (w293:dbl)
                              n474 = Subtract(x=w293, y=2.0) -> (x-y=w292:dbl)
                              n475 = local write "Production Tank"(w292) -> ()
                              n476 = local read "Production Tank"() -> (w288:dbl)
                              n477 = local read "bottels ready"() -> (w284:dbl)
                              n478 = Less?(x=w288, y=2.0) -> (x < y?=w287:bool)
                              n479 = Add(x=w284, y=0.67) -> (x+y=w285:dbl)
                              n480 = local write "bottels ready"(w285) -> ()
                            }
                          }
                          frame True {
                            n481 = property on="Boolean 5" class="Bool (strict)"("Visible"=TRUE) -> ()  [unwired: 2 in, 2 out]
                            n482 = property on="Boolean" class="Bool (strict)"("Visible"=TRUE) -> ()  [unwired: 2 in, 2 out]
                            n483 = property on="Boolean 2" class="Bool (strict)"("Visible"=TRUE) -> ()  [unwired: 2 in, 2 out]
                            n484 = property on="Boolean 4" class="Bool (strict)"("Visible"=TRUE) -> ()  [unwired: 2 in, 2 out]
                            n485 = property on="Boolean 3" class="Bool (strict)"("Visible"=TRUE) -> ()  [unwired: 2 in, 2 out]
                            n486 = while {
                              stop <- w306 stop-if-true
                              n487 = flat-sequence {
                                frame #0 {
                                n488 = local write "Boolean 5"(TRUE ("Boolean 5")) -> ()
                                n489 = Wait (ms)(milliseconds to wait=u32 500) -> ()  [unwired: 1 out]
                                }
                                frame #1 {
                                w318 = TRUE ("Boolean 3")
                                n490 = local write "Boolean 4"(w318) -> ()
                                n491 = local write "Boolean 3"(w318) -> ()
                                n492 = Wait (ms)(milliseconds to wait=u32 500) -> ()  [unwired: 1 out]
                                }
                                frame #2 {
                                w320 = TRUE ("Boolean")
                                n493 = local write "Boolean 2"(w320) -> ()
                                n494 = local write "Boolean"(w320) -> ()
                                n495 = Wait (ms)(milliseconds to wait=u32 500) -> ()  [unwired: 1 out]
                                }
                                frame #3 {
                                n496 = local write "Boolean 5"(FALSE ("Boolean 5")) -> ()
                                }
                                frame #4 {
                                w322 = FALSE ("Boolean 3")
                                n497 = local write "Boolean 4"(w322) -> ()
                                n498 = local write "Boolean 3"(w322) -> ()
                                }
                                frame #5 {
                                w323 = FALSE ("Boolean")
                                n499 = local write "Boolean 2"(w323) -> ()
                                n500 = local write "Boolean"(w323) -> ()
                                }
                              }
                              n501 = Wait (ms)(milliseconds to wait=u32 1000) -> ()  [unwired: 1 out]
                              n502 = local read "Production Tank"() -> (w314:dbl)
                              n503 = Subtract(x=w314, y=2.0) -> (x-y=w313:dbl)
                              n504 = local write "Production Tank"(w313) -> ()
                              n505 = local read "bottels ready"() -> (w310:dbl)
                              n506 = local read "Production Tank"() -> (w305:dbl)
                              n507 = Add(x=w310, y=0.4) -> (x+y=w309:dbl)
                              n508 = Less?(x=w305, y=2.0) -> (x < y?=w306:bool)
                              n509 = local write "bottels ready"(w309) -> ()
                            }
                          }
                        }
                        n510 = property on="bottels ready" class="Slide (strict)"("Visible"=TRUE) -> ()  [unwired: 2 in, 2 out]
                        n511 = local write "status"("Filling Bottels" ("status")) -> ()
                        n512 = property on="Classifier material" class="Slide (strict)"("Visible"=FALSE) -> ()  [unwired: 2 in, 2 out]
                        n513 = property on="Water" class="Slide (strict)"("Visible"=FALSE) -> ()  [unwired: 2 in, 2 out]
                        n514 = property on="Virus A" class="Slide (strict)"("Visible"=FALSE) -> ()  [unwired: 2 in, 2 out]
                        n515 = property on="Virus B" class="Slide (strict)"("Visible"=FALSE) -> ()  [unwired: 2 in, 2 out]
                        n516 = property on="Virus C" class="Slide (strict)"("Visible"=FALSE) -> ()  [unwired: 2 in, 2 out]
                      }
                      frame #16 {
                        n517 = local read "Classifier material"() -> (w328:dbl)
                        n518 = local read "Virus B"() -> (w325:dbl)
                        n519 = local read "Virus C"() -> (w324:dbl)
                        n520 = local read "Water"() -> (w327:dbl)
                        n521 = local read "Virus A"() -> (w326:dbl)
                        n522 = local write "EXIT"(TRUE ("EXIT")) -> ()
                        n523 = local write "v ok"(TRUE ("v ok")) -> ()
                        n524 = global write "Global 3.vi" "Classifier material"(w328) -> ()
                        n525 = global write "Global 3.vi" "Virus B"(w325) -> ()
                        n526 = global write "Global 3.vi" "Virus A"(w326) -> ()
                        n527 = global write "Global 3.vi" "Virus C"(w324) -> ()
                        n528 = global write "Global 3.vi" "Water"(w327) -> ()
                      }
                    }
                  }
                }
                n529 = case shown="True" w142 {
                  frame False {
                  }
                  frame True {
                    n530 = flat-sequence {
                      frame #0 {
                        n531 = property on="Production Tank" class="Slide (strict)"("Visible"=TRUE) -> ()  [unwired: 2 in, 2 out]
                        n532 = local write "start"(FALSE ("start")) -> ()
                        n533 = property on="start" class="Bool (strict)"("Visible"=FALSE) -> ()  [unwired: 2 in, 2 out]
                      }
                      frame #1 {
                        n534 = local read "ML INT"() -> (w527:dbl)
                        n535 = Multiply(x=0.05 ("y"), y=w527) -> (x*y=w528:dbl)
                        n536 = local read "camot"() -> (w525:dbl)
                        n537 = Multiply(x=w525, y=w528) -> (x*y=w524:dbl)
                        n538 = Divide(x=w524, y=2.0) -> (x/y=→"x/y":dbl)
                      }
                      frame #2 {
                        n539 = local read "x/y"() -> (w530:dbl)
                        n540 = Round Toward -Infinity(1:w530) -> (0:→"N itertion":dbl)
                      }
                      frame #3 {
                        n541 = local read "N itertion"() -> (w531:dbl)
                        n542 = Multiply(x=w531, y=2.0) -> (x*y=→"int":dbl)
                      }
                      frame #4 {
                        n543 = local read "N itertion"() -> (w534:dbl)
                        n544 = for {
                          N: w534 -> [_]
                          n545 = local read "Classifier material"() -> (w542:dbl)
                          n546 = local read "Production Tank"() -> (w540:dbl)
                          n547 = Wait (ms)(milliseconds to wait=u32 1000) -> ()  [unwired: 1 out]
                          n548 = Add(x=w540, y=2.0) -> (x+y=w539:dbl)
                          n549 = Subtract(x=w542, y=2.0) -> (x-y=w541:dbl)
                          n550 = local write "Production Tank"(w539) -> ()
                          n551 = local write "Classifier material"(w541) -> ()
                          n552 = local write "status"("Addind Classified material" ("status")) -> ()
                        }
                      }
                      frame #5 {
                        n553 = local read "ML INT"() -> (w546:dbl)
                        n554 = local read "ML INT"() -> (w547:dbl)
                        n555 = local write "status"("Addind Classified material" ("status")) -> ()
                        n556 = Multiply(x=0.05 ("y"), y=w546) -> (x*y=w544:dbl)
                        n557 = Multiply(x=0.05 ("y"), y=w547) -> (x*y=w543:dbl)
                        n558 = local read "camot"() -> (w560:dbl)
                        n559 = local read "camot"() -> (w553:dbl)
                        n560 = Multiply(x=w560, y=w544) -> (x*y=w559:dbl)
                        n561 = Multiply(x=w553, y=w543) -> (x*y=w552:dbl)
                        n562 = local read "int"() -> (w558:dbl)
                        n563 = local read "int"() -> (w551:dbl)
                        n564 = Subtract(x=w559, y=w558) -> (x-y=w557:dbl)
                        n565 = Subtract(x=w552, y=w551) -> (x-y=w554:dbl)
                        n566 = local read "Classifier material"() -> (w561:dbl)
                        n567 = local read "Production Tank"() -> (w555:dbl)
                        n568 = Subtract(x=w561, y=w557) -> (x-y=w562:dbl)
                        n569 = Add(x=w555, y=w554) -> (x+y=w556:dbl)
                        n570 = local write "Classifier material"(w562) -> ()
                        n571 = local write "Production Tank"(w556) -> ()
                        n572 = Wait (ms)(milliseconds to wait=u32 1000) -> ()  [unwired: 1 out]
                      }
                      frame #6 {
                        n573 = local read "ML INT"() -> (w564:dbl)
                        n574 = Multiply(x=w564, y=0.22) -> (x*y=w563:dbl)
                        n575 = local read "camot"() -> (w569:dbl)
                        n576 = Multiply(x=w569, y=w563) -> (x*y=w568:dbl)
                        n577 = Divide(x=w568, y=2.0) -> (x/y=→"x/y 2":dbl)
                      }
                      frame #7 {
                        n578 = local read "x/y 2"() -> (w571:dbl)
                        n579 = Round Toward -Infinity(1:w571) -> (0:→"N itertion 2":dbl)
                      }
                      frame #8 {
                        n580 = local read "N itertion 2"() -> (w572:dbl)
                        n581 = Multiply(x=w572, y=2.0) -> (x*y=→"int 2":dbl)
                      }
                      frame #9 {
                        n582 = local read "N itertion 2"() -> (w575:dbl)
                        n583 = for {
                          N: w575 -> [_]
                          n584 = local read "Water"() -> (w582:dbl)
                          n585 = Wait (ms)(milliseconds to wait=u32 1000) -> ()  [unwired: 1 out]
                          n586 = local read "Production Tank"() -> (w576:dbl)
                          n587 = Subtract(x=w582, y=2.0) -> (x-y=w583:dbl)
                          n588 = local write "Water"(w583) -> ()
                          n589 = local write "status"("Addind Water" ("status")) -> ()
                          n590 = Add(x=w576, y=2.0) -> (x+y=w577:dbl)
                          n591 = local write "Production Tank"(w577) -> ()
                        }
                      }
                      frame #10 {
                        n592 = local read "ML INT"() -> (w587:dbl)
                        n593 = local read "ML INT"() -> (w589:dbl)
                        n594 = Multiply(x=w587, y=0.22) -> (x*y=w584:dbl)
                        n595 = Multiply(x=w589, y=0.22) -> (x*y=w585:dbl)
                        n596 = local read "camot"() -> (w599:dbl)
                        n597 = local read "camot"() -> (w594:dbl)
                        n598 = Multiply(x=w599, y=w584) -> (x*y=w600:dbl)
                        n599 = Multiply(x=w594, y=w585) -> (x*y=w595:dbl)
                        n600 = local read "int 2"() -> (w598:dbl)
                        n601 = local read "int 2"() -> (w590:dbl)
                        n602 = Subtract(x=w600, y=w598) -> (x-y=w601:dbl)
                        n603 = Subtract(x=w595, y=w590) -> (x-y=w593:dbl)
                        n604 = local read "Production Tank"() -> (w592:dbl)
                        n605 = local read "Water"() -> (w596:dbl)
                        n606 = Subtract(x=w596, y=w601) -> (x-y=w597:dbl)
                        n607 = Add(x=w592, y=w593) -> (x+y=w591:dbl)
                        n608 = local write "Production Tank"(w591) -> ()
                        n609 = local write "Water"(w597) -> ()
                        n610 = Wait (ms)(milliseconds to wait=u32 1000) -> ()  [unwired: 1 out]
                      }
                      frame #11 {
                        n611 = local read "ML INT"() -> (w604:dbl)
                        n612 = Multiply(x=w604, y=0.73) -> (x*y=w603:dbl)
                        n613 = local read "camot"() -> (w609:dbl)
                        n614 = Multiply(x=w609, y=w603) -> (x*y=w608:dbl)
                        n615 = Divide(x=w608, y=2.0) -> (x/y=→"x/y 3":dbl)
                      }
                      frame #12 {
                        n616 = local read "x/y 3"() -> (w611:dbl)
                        n617 = Round Toward -Infinity(1:w611) -> (0:→"N itertion 3":dbl)
                      }
                      frame #13 {
                        n618 = local read "N itertion 3"() -> (w612:dbl)
                        n619 = Multiply(x=w612, y=2.0) -> (x*y=→"int 3":dbl)
                      }
                      frame #14 {
                        n620 = local read "N itertion 3"() -> (w615:dbl)
                        n621 = for {
                          N: w615 -> [_]
                          n622 = local read "Virus A"() -> (w622:dbl)
                          n623 = local read "Production Tank"() -> (w617:dbl)
                          n624 = Wait (ms)(milliseconds to wait=u32 1000) -> ()  [unwired: 1 out]
                          n625 = Subtract(x=w622, y=2.0) -> (x-y=w620:dbl)
                          n626 = local write "status"("Addind Virus A" ("status")) -> ()
                          n627 = local write "Virus A"(w620) -> ()
                          n628 = Add(x=w617, y=2.0) -> (x+y=w618:dbl)
                          n629 = local write "Production Tank"(w618) -> ()
                        }
                      }
                      frame #15 {
                        n630 = local read "ML INT"() -> (w626:dbl)
                        n631 = local read "ML INT"() -> (w629:dbl)
                        n632 = Multiply(x=w626, y=0.73) -> (x*y=w624:dbl)
                        n633 = Multiply(x=w629, y=0.73) -> (x*y=w627:dbl)
                        n634 = local read "camot"() -> (w639:dbl)
                        n635 = local read "camot"() -> (w637:dbl)
                        n636 = Multiply(x=w639, y=w624) -> (x*y=w638:dbl)
                        n637 = Multiply(x=w637, y=w627) -> (x*y=w636:dbl)
                        n638 = local read "int 3"() -> (w630:dbl)
                        n639 = local read "int 3"() -> (w631:dbl)
                        n640 = Subtract(x=w638, y=w630) -> (x-y=w640:dbl)
                        n641 = Subtract(x=w636, y=w631) -> (x-y=w635:dbl)
                        n642 = local read "Production Tank"() -> (w641:dbl)
                        n643 = local read "Virus A"() -> (w632:dbl)
                        n644 = Add(x=w641, y=w640) -> (x+y=w642:dbl)
                        n645 = Subtract(x=w632, y=w635) -> (x-y=w633:dbl)
                        n646 = local write "Production Tank"(w642) -> ()
                        n647 = local write "Virus A"(w633) -> ()
                        n648 = Wait (ms)(milliseconds to wait=u32 1000) -> ()  [unwired: 1 out]
                      }
                      frame #16 {
                        n649 = Wait (ms)(milliseconds to wait=u32 17000) -> ()  [unwired: 1 out]
                        n650 = property on="Production Tank" class="Slide (strict)"("Blinking"=TRUE) -> ()  [unwired: 2 in, 2 out]
                        n651 = local write "status"("Quality Control" ("status")) -> ()
                      }
                      frame #17 {
                        n652 = local read "ML INT"() -> (w648:dbl)
                        n653 = local write "status"("Filling Bottels" ("status")) -> ()
                        n654 = property on="Production Tank" class="Slide (strict)"("Blinking"=FALSE) -> ()  [unwired: 2 in, 2 out]
                        n655 = Equal?(x=w648, y=5.0) -> (x = y?=w646:bool)
                        n656 = property on="bottels ready" class="Slide (strict)"("Visible"=TRUE) -> ()  [unwired: 2 in, 2 out]
                        n657 = case shown="True" w646 {
                          frame False {
                            n658 = property on="Boolean" class="Bool (strict)"("Visible"=TRUE) -> ()  [unwired: 2 in, 2 out]
                            n659 = property on="Boolean 2" class="Bool (strict)"("Visible"=TRUE) -> ()  [unwired: 2 in, 2 out]
                            n660 = property on="Boolean 3" class="Bool (strict)"("Visible"=TRUE) -> ()  [unwired: 2 in, 2 out]
                            n661 = while {
                              stop <- w660 stop-if-true
                              n662 = flat-sequence {
                                frame #0 {
                                n663 = local write "Boolean 3"(TRUE ("Boolean 3")) -> ()
                                n664 = Wait (ms)(milliseconds to wait=u32 1000) -> ()  [unwired: 1 out]
                                }
                                frame #1 {
                                w673 = TRUE ("Boolean")
                                n665 = local read "bottels ready"() -> (w671:dbl)
                                n666 = Wait (ms)(milliseconds to wait=u32 1000) -> ()  [unwired: 1 out]
                                n667 = Add(x=w671, y=1.0) -> (x+y=w670:dbl)
                                n668 = local write "bottels ready"(w670) -> ()
                                n669 = local write "Boolean 2"(w673) -> ()
                                n670 = local write "Boolean"(w673) -> ()
                                }
                                frame #2 {
                                n671 = local write "Boolean 3"(FALSE ("Boolean 3")) -> ()
                                }
                                frame #3 {
                                w675 = FALSE ("Boolean")
                                n672 = local write "Boolean 2"(w675) -> ()
                                n673 = local write "Boolean"(w675) -> ()
                                }
                              }
                              n674 = Wait (ms)(milliseconds to wait=u32 1000) -> ()  [unwired: 1 out]
                              n675 = local read "Production Tank"() -> (w666:dbl)
                              n676 = Subtract(x=w666, y=2.0) -> (x-y=w665:dbl)
                              n677 = local write "Production Tank"(w665) -> ()
                              n678 = local read "Production Tank"() -> (w661:dbl)
                              n679 = Less?(x=w661, y=2.0) -> (x < y?=w660:bool)
                            }
                          }
                          frame True {
                            n680 = property on="Boolean 5" class="Bool (strict)"("Visible"=TRUE) -> ()  [unwired: 2 in, 2 out]
                            n681 = property on="Boolean" class="Bool (strict)"("Visible"=TRUE) -> ()  [unwired: 2 in, 2 out]
                            n682 = property on="Boolean 2" class="Bool (strict)"("Visible"=TRUE) -> ()  [unwired: 2 in, 2 out]
                            n683 = property on="Boolean 4" class="Bool (strict)"("Visible"=TRUE) -> ()  [unwired: 2 in, 2 out]
                            n684 = property on="Boolean 3" class="Bool (strict)"("Visible"=TRUE) -> ()  [unwired: 2 in, 2 out]
                            n685 = while {
                              stop <- w682 stop-if-true
                              n686 = flat-sequence {
                                frame #0 {
                                n687 = local write "Boolean 5"(TRUE ("Boolean 5")) -> ()
                                n688 = Wait (ms)(milliseconds to wait=u32 500) -> ()  [unwired: 1 out]
                                }
                                frame #1 {
                                w694 = TRUE ("Boolean 3")
                                n689 = local write "Boolean 4"(w694) -> ()
                                n690 = local write "Boolean 3"(w694) -> ()
                                n691 = Wait (ms)(milliseconds to wait=u32 500) -> ()  [unwired: 1 out]
                                }
                                frame #2 {
                                w696 = TRUE ("Boolean")
                                n692 = local write "Boolean 2"(w696) -> ()
                                n693 = local write "Boolean"(w696) -> ()
                                n694 = Wait (ms)(milliseconds to wait=u32 500) -> ()  [unwired: 1 out]
                                }
                                frame #3 {
                                n695 = local write "Boolean 5"(FALSE ("Boolean 5")) -> ()
                                }
                                frame #4 {
                                w698 = FALSE ("Boolean 3")
                                n696 = local write "Boolean 4"(w698) -> ()
                                n697 = local write "Boolean 3"(w698) -> ()
                                }
                                frame #5 {
                                w699 = FALSE ("Boolean")
                                n698 = local write "Boolean 2"(w699) -> ()
                                n699 = local write "Boolean"(w699) -> ()
                                }
                              }
                              n700 = Wait (ms)(milliseconds to wait=u32 1000) -> ()  [unwired: 1 out]
                              n701 = local read "Production Tank"() -> (w690:dbl)
                              n702 = Subtract(x=w690, y=2.0) -> (x-y=w689:dbl)
                              n703 = local write "Production Tank"(w689) -> ()
                              n704 = local read "bottels ready"() -> (w686:dbl)
                              n705 = local read "Production Tank"() -> (w681:dbl)
                              n706 = Add(x=w686, y=0.4) -> (x+y=w685:dbl)
                              n707 = Less?(x=w681, y=2.0) -> (x < y?=w682:bool)
                              n708 = local write "bottels ready"(w685) -> ()
                            }
                          }
                        }
                        n709 = property on="Classifier material" class="Slide (strict)"("Visible"=FALSE) -> ()  [unwired: 2 in, 2 out]
                        n710 = property on="Water" class="Slide (strict)"("Visible"=FALSE) -> ()  [unwired: 2 in, 2 out]
                        n711 = property on="Virus A" class="Slide (strict)"("Visible"=FALSE) -> ()  [unwired: 2 in, 2 out]
                        n712 = property on="Virus B" class="Slide (strict)"("Visible"=FALSE) -> ()  [unwired: 2 in, 2 out]
                        n713 = property on="Virus C" class="Slide (strict)"("Visible"=FALSE) -> ()  [unwired: 2 in, 2 out]
                      }
                      frame #18 {
                        n714 = local read "Virus B"() -> (w703:dbl)
                        n715 = local read "Classifier material"() -> (w705:dbl)
                        n716 = local read "Virus C"() -> (w704:dbl)
                        n717 = local read "Virus A"() -> (w701:dbl)
                        n718 = local read "Water"() -> (w702:dbl)
                        n719 = global write "Global 3.vi" "Virus B"(w703) -> ()
                        n720 = global write "Global 3.vi" "Virus C"(w704) -> ()
                        n721 = global write "Global 3.vi" "Virus A"(w701) -> ()
                        n722 = global write "Global 3.vi" "Water"(w702) -> ()
                        n723 = global write "Global 3.vi" "Classifier material"(w705) -> ()
                        n724 = local write "v ok"(TRUE ("v ok")) -> ()
                        n725 = local write "EXIT"(TRUE ("EXIT")) -> ()
                      }
                    }
                  }
                }
              }
            }
          }
        }
        "status" <- " " ("status")
        "Production Tank" <- 0.0 ("Production Tank")
        "bottels ready" <- 0.0 ("bottels ready")
      }
    }
    frame #2 {
      n726 = local read "Virus B"() -> (w711:dbl)
      n727 = global write "Global 3.vi" "Virus B"(w711) -> ()
      n728 = local read "Virus C"() -> (w710:dbl)
      n729 = local read "Water"() -> (w708:dbl)
      n730 = local read "Classifier material"() -> (w707:dbl)
      n731 = global write "Global 3.vi" "Classifier material"(w707) -> ()
      n732 = global write "Global 3.vi" "Virus C"(w710) -> ()
      n733 = global write "Global 3.vi" "Water"(w708) -> ()
      n734 = local read "Virus A"() -> (w709:dbl)
      n735 = global write "Global 3.vi" "Virus A"(w709) -> ()
    }
    frame #3 {
      n736 = local read "v ok"() -> (w712:bool)
      n737 = case shown="True" w712 {
        frame False {
        }
        frame True {
          n738 = flat-sequence {
            frame #0 {
              n739 = local read "row"() -> (w713:i32)
              n740 = for {
                N: w713 -> [w723]
                tunnel: [w723] -> _ mode=indexing
                i -> [w715]
                n741 = local read "orders"() -> (w722:string[][])
                n742 = local read "Order"() -> (w720:string[])
                n743 = Index Array(array=w722, index (row)=w715, index (col)=0 ("disabled index (col)")) -> (element=w718:string)
                "element" <- w718
                n744 = Index Array(array=w720, index=0) -> (element=w717:string)
                "element 2" <- w717
                n745 = Equal?(x=w718, y=w717) -> (x = y?=w716:bool)
                n746 = case shown="True" w716 {
                  tunnel: w715 -> [_ w725]
                  frame False {
                  }
                  frame True {
                    n747 = local read "orders"() -> (w724:string[][])
                    n748 = Delete From Array(array=w724, index (row)=w725) -> (array with subset deleted=w726:string[][])  [unwired: 2 in, 1 out]
                    n749 = local write "orders"(w726) -> ()
                  }
                }
              }
              n750 = local write "v ok"(FALSE ("v ok")) -> ()
            }
            frame #1 {
              n751 = Current VI's Path() -> (path=w727:path)
              n752 = local read "orders"() -> (w733:string[][])
              n753 = Strip Path(path=w727) -> (stripped path=w728:path)  [unwired: 1 out]
              n754 = Build Path(base path=w728, name or relative path="order list.xls") -> (appended path=w729:path)
              n755 = call-poly <vilib>:"Write To Spreadsheet File.vi"("transpose? (no:F)"=FALSE, "append to file? (new file:F)"=FALSE, "2D data"=w733, "file path (dialog if empty)"=w729) -> ()  [unwired: 4 in, 1 out]
            }
            frame #2 {
              n756 = call "Display Message to User5"() -> ()  [unwired: 10 in, 2 out]
            }
          }
        }
      }
    }
    frame #4 {
      n757 = flat-sequence {
        frame #0 {
          n758 = Current VI's Path() -> (path=w737:path)
          n759 = Open VI Reference(vi path=w737) -> (error out=w736:errorcluster)  [unwired: 5 in, 1 out]
          n760 = invoke class="VI" method="FP.Close"(error in=w736) -> (reference out=w734:refnum<vi>, error out=w735:errorcluster)  [unwired: 2 in, 1 out]
          n761 = Close Reference(reference=w734, error in (no error)=w735) -> ()  [unwired: 1 out]
        }
      }
    }
  }
